vi "Disable During Save (SubVI).vi"(7 "References":T1) -> ()   [LabVIEW 2010]
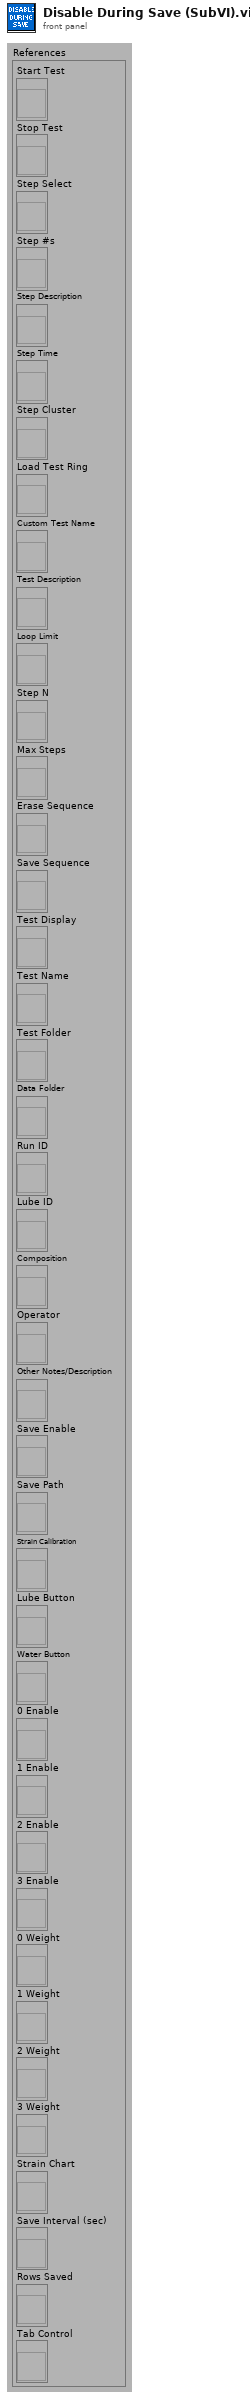
[diagram p1: front panel]
types:
  T1 = cluster{"Start Test":refnum<vi>, "Stop Test":refnum<vi>, "Step Select":refnum<vi>, "Step #s":refnum<vi>, "Step Description":refnum<vi>, "Step Time":refnum<vi>, "Step Cluster":refnum<vi>, "Load Test Ring":refnum<vi>, "Custom Test Name":refnum<vi>, "Test Description":refnum<vi>, "Loop Limit":refnum<vi>, "Step N":refnum<vi>, "Max Steps":refnum<vi>, "Erase Sequence":refnum<vi>, "Save Sequence":refnum<vi>, "Test Display":refnum<vi>, "Test Name":refnum<vi>, "Test Folder":refnum<vi>, "Data Folder":refnum<vi>, "Run ID":refnum<vi>, "Lube ID":refnum<vi>, "Composition":refnum<vi>, "Operator":refnum<vi>, "Other Notes/Description":refnum<vi>, "Save Enable":refnum<vi>, "Save Path":refnum<vi>, "Strain Calibration":refnum<vi>, "Lube Button":refnum<vi>, "Water Button":refnum<vi>, "0 Enable":refnum<vi>, "1 Enable":refnum<vi>, "2 Enable":refnum<vi>, "3 Enable":refnum<vi>, "0 Weight":refnum<vi>, "1 Weight":refnum<vi>, "2 Weight":refnum<vi>, "3 Weight":refnum<vi>, "Strain Chart":refnum<vi>, "Save Interval (sec)":refnum<vi>, "Rows Saved":refnum<vi>, "Tab Control":refnum<vi>}
  T2 = enum8{"Enabled", "Disabled", "Disabled and Grayed Out"}
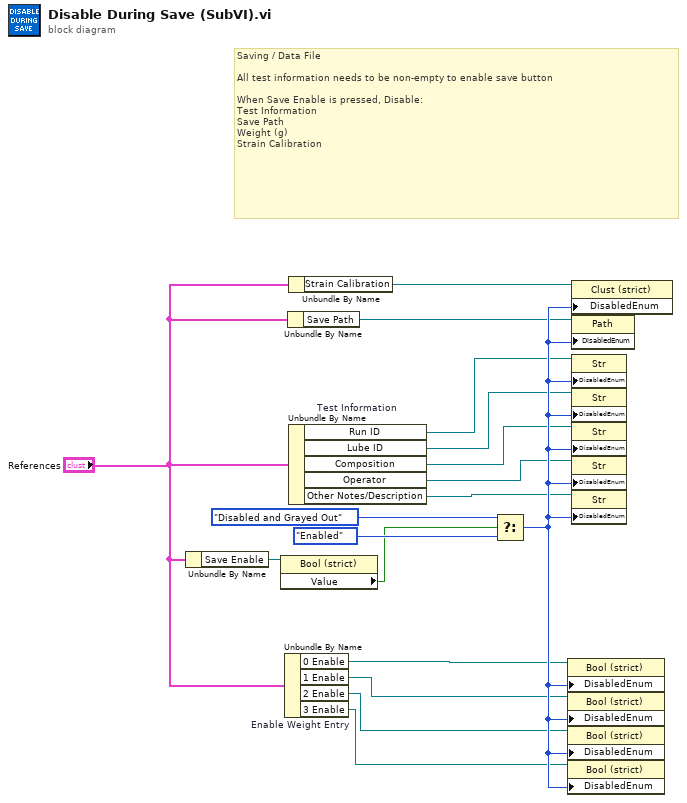
[diagram p0: block diagram]
diagram:
  # "Saving / Data File\n\nAll test information needs to be non-empty to enable save button\n\nWhen Save Enable is pressed, Disable:\nTest Information\nSave Path\nWeight (g)\nStrain Calibration"
  n1 = Unbundle By Name("References") -> ("Save Enable"=w10:refnum<vi>)
  n2 = property class="Bool (strict)"(reference=w10) -> ("Value"=w2:bool)  [unwired: 1 in, 2 out]
  n3 = Unbundle By Name "Enable Weight Entry"("References") -> ("0 Enable"=w11:refnum<vi>, "1 Enable"=w12:refnum<vi>, "2 Enable"=w13:refnum<vi>, "3 Enable"=w14:refnum<vi>)
  n4 = Unbundle By Name("References") -> ("Save Path"=w4:refnum<vi>)
  n5 = Unbundle By Name("References") -> ("Strain Calibration"=w5:refnum<vi>)
  n6 = Unbundle By Name "Test Information"("References") -> ("Run ID"=w6:refnum<vi>, "Lube ID"=w7:refnum<vi>, "Composition"=w8:refnum<vi>, "Operator"=w9:refnum<vi>, "Other Notes/Description"=w3:refnum<vi>)
  n7 = Select(t=T2."Disabled and Grayed Out" ("Disabled"), s=w2, f=T2."Enabled" ("Disabled")) -> (s? t:f=w16:T2)
  n8 = property class="Bool (strict)"(reference=w11, "DisabledEnum"=w16) -> ()  [unwired: 1 in, 2 out]
  n9 = property class="Bool (strict)"(reference=w12, "DisabledEnum"=w16) -> ()  [unwired: 1 in, 2 out]
  n10 = property class="Bool (strict)"(reference=w13, "DisabledEnum"=w16) -> ()  [unwired: 1 in, 2 out]
  n11 = property class="Bool (strict)"(reference=w14, "DisabledEnum"=w16) -> ()  [unwired: 1 in, 2 out]
  n12 = property class="Clust (strict)"(reference=w5, "DisabledEnum"=w16) -> ()  [unwired: 1 in, 2 out]
  n13 = property class="Path"(reference=w4, "DisabledEnum"=w16) -> ()  [unwired: 1 in, 2 out]
  n14 = property class="Str"(reference=w6, "DisabledEnum"=w16) -> ()  [unwired: 1 in, 2 out]
  n15 = property class="Str"(reference=w7, "DisabledEnum"=w16) -> ()  [unwired: 1 in, 2 out]
  n16 = property class="Str"(reference=w8, "DisabledEnum"=w16) -> ()  [unwired: 1 in, 2 out]
  n17 = property class="Str"(reference=w9, "DisabledEnum"=w16) -> ()  [unwired: 1 in, 2 out]
  n18 = property class="Str"(reference=w3, "DisabledEnum"=w16) -> ()  [unwired: 1 in, 2 out]
